vi "LDR VTH 2 LEDS.vi"() -> ()   [LabVIEW 2017]
uses:
  <vilib>/MakerHub/LINX/Public/Peripherals/Digital/Digital Read 1 Chan.vi
  <vilib>/MakerHub/LINX/Public/Peripherals/Digital/Digital Write 1 Chan.vi
  <vilib>/MakerHub/LINX/Public/Peripherals/Digital/Digital Read N Chans.vi
  <vilib>/MakerHub/LINX/Public/Peripherals/Digital/Digital Write N Chans.vi
  <vilib>/MakerHub/LINX/Private/Local IO/LinxDigitalRead.vi
  <vilib>/MakerHub/LINX/Public/Utilities/Check Channel.vi
  <vilib>/MakerHub/LINX/Private/Local IO/LinxDigitalWrite.vi
  <vilib>/MakerHub/LINX/Public/Utilities/Open Serial.vi
  <vilib>/MakerHub/LINX/Private/Utilties/Generate Error.vi
  <vilib>/MakerHub/LINX/LMH-LINX.lvlib
panel:
  in  "DO Channel 2":u8
  in  "DO Channel":u8
  in  "DI Channel":u8
  out "DI Value":bool
  in  "stop":bool
  in  "Serial Port":refnum<visa-resource-name>="N/A"
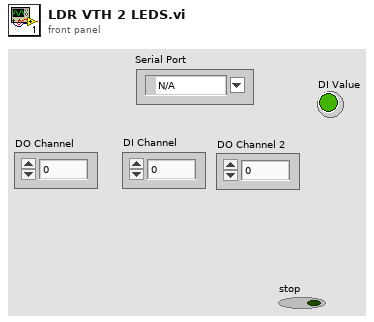
[diagram p1: front panel]
types:
  T1 = typedef "LMH-LINX.lvlib/LINX Ref.ctl" = cluster{"IO":T2, "Interface":T3, "LINX Device Config":T4}
  T2 = typedef "LMH-LINX.lvlib/Platform.ctl" = enum16{"Remote", "Local"}
  T3 = typedef "LMH-LINX.lvlib/Interface.ctl" = enum16{"Serial", "TCP"}
  T4 = typedef "LMH-LINX.lvlib/Device.lvlib/LINX Device Config.ctl" = cluster{"Interface":T3, "COM Port":refnum<visa-resource-name>, "TCP Configuration":T5, "Device Family":u8, "Device ID":u8, "Device Name":string, "TCP Ref":refnum<k5>, "Channels":T6}
  T5 = typedef "LMH-LINX.lvlib/Device.lvlib/TCP Config.ctl" = cluster{"IP Address":string, "Port":u16}
  T6 = typedef "LMH-LINX.lvlib/Channels.ctl" = cluster{"DI":u8[], "DO":u8[], "AI":u8[], "AO":u8[], "PWM":u8[], "QE":u8[], "UART":u8[], "I2C 2":u8[], "SPI":u8[], "CAN":u8[], "Servo":u8[], "AI Ref (V)":dbl, "AI Resolution (Bits)":u8, "AO Ref (V)":dbl, "AO Resolution (Bits)":u8}
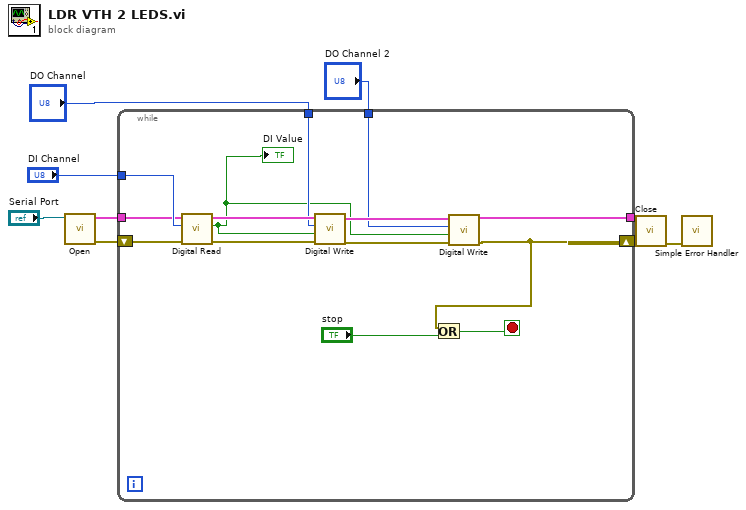
[diagram p0: block diagram]
diagram:
  n1 = call-poly <vilib>:"Open.vi"("Serial Port"="Serial Port") -> ("Error Out"=w7:errorcluster, "LINX Resource"=w8:T1)  [unwired: 8 in, 1 out]
  n2 = while {
    tunnel: w8 -> [w20]
    shift-right: [w12] -> w5
    shift-left: w7 -> [w18]
    tunnel: "DI Channel" -> [w21]
    tunnel: [w14] -> w3
    tunnel: "DO Channel" -> [w16]
    tunnel: "DO Channel 2" -> [w11]
    stop <- w23 stop-if-true
    n3 = call-poly <vilib>:"Digital Read.vi"("Error In"=w18, "DI Channel"=w21, "LINX Resource"=w20) -> ("Error Out"=w17:errorcluster, "DI Value"=w10:bool, "LINX Resource"=w19:T1)  [unwired: 6 in]
    "DI Value" <- w10
    n4 = call-poly <vilib>:"Digital Write.vi"("Error In"=w17, "Output Value"=w10, "DO Channel"=w16, "LINX Resource"=w19) -> ("Error Out"=w13:errorcluster, "LINX Resource"=w15:T1)  [unwired: 6 in]
    n5 = call-poly <vilib>:"Digital Write.vi"("Error In"=w13, "Output Value"=w10, "DO Channel"=w11, "LINX Resource"=w15) -> ("Error Out"=w12:errorcluster, "LINX Resource"=w14:T1)  [unwired: 6 in]
    n6 = Or(x=w12, y="stop") -> (x .or. y?=w23:bool)
  }
  n7 = call <vilib>:"Close.vi"("Error In"=w5, "LINX Resource"=w3) -> ("Error Out"=w6:errorcluster)  [unwired: 9 in]
  n8 = call <vilib>:"Simple Error Handler.vi"("error in (no error)"=w6) -> ()  [unwired: 4 in, 5 out]
